vi "Find Center Setup.vi"(0 "Carrier Tray":T1, 1 "Tray Number":dbl format="%#_13g") -> (7 "Assembly Tray Out":T1)   [LabVIEW 2019, in "Assembly Tray.lvclass"]
uses:
  Assembly Tray.lvclass
  Find Tray.ctl
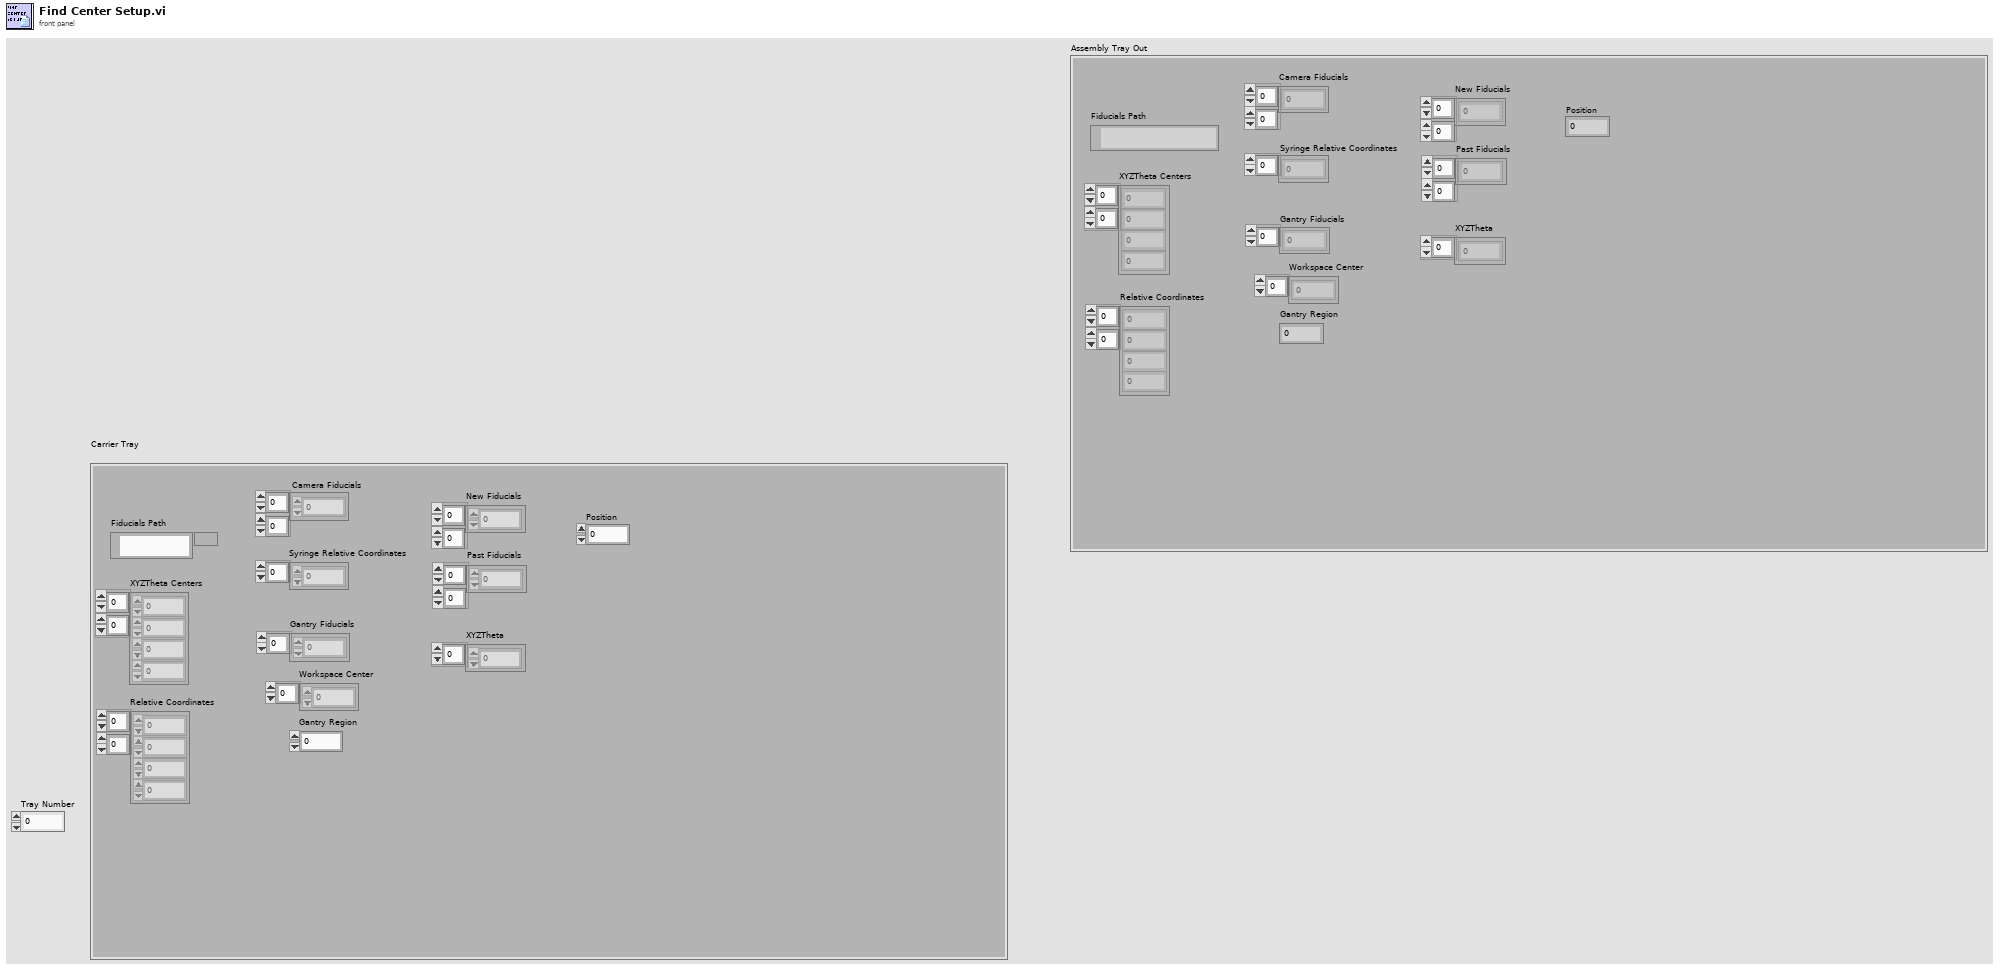
[diagram p1: front panel]
types:
  T1 = typedef "Assembly Tray.lvclass/Find Tray.ctl" = cluster{"Gantry Fiducials":dbl[], "Relative Coordinates":dbl[][], "Camera Fiducials":dbl[][], "XYZTheta Centers":dbl[][], "Workspace Center":dbl[], "Syringe Relative Coordinates":dbl[], "Gantry Region":dbl, "Fiducials Path":path, "New Fiducials":dbl[][], "Past Fiducials":dbl[][], "XYZTheta":dbl[], "Position":i32}
  T2 = typedef "File Paths.ctl" = cluster{"Glue Pattern Folder":path, "Carrier Tray Folder":path, "Pick Up Tool Fixture Folder":path, "Components Folder":path, "Bellows Tool Offset.txt":path, "Pick Up Tool Offset.txt":path, "Dispense Tip Offset.txt":path, "Log Files":path}
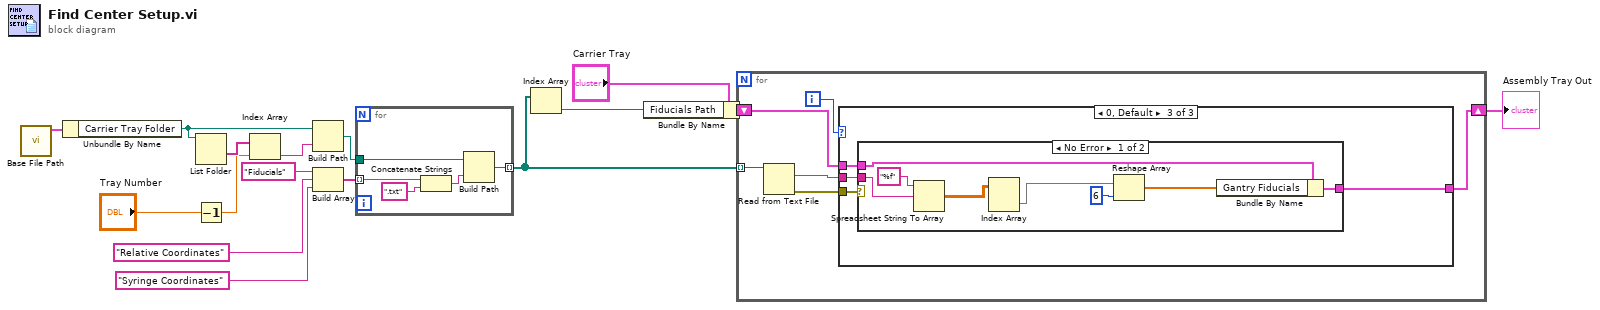
[diagram p0: block diagram]
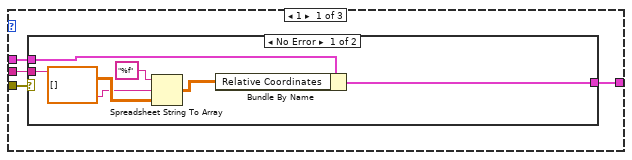
[diagram p2: hidden frame]
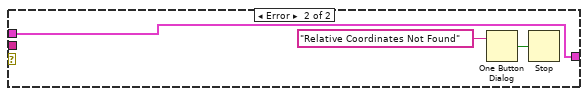
[diagram p3: hidden frame]
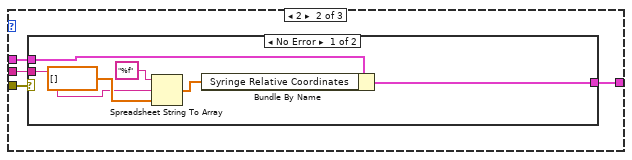
[diagram p4: hidden frame]
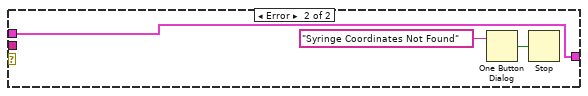
[diagram p5: hidden frame]
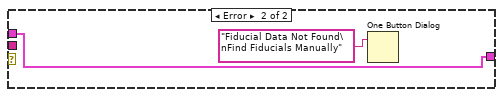
[diagram p6: hidden frame]
diagram:
  n1 = call "Base File Path.vi"() -> ("Paths Out"=w8:T2)  [unwired: 11 in]
  n2 = Unbundle By Name(w8) -> ("Carrier Tray Folder"=w4:path)
  n3 = List Folder(path=w4) -> (folder names=w10:string[])  [unwired: 3 in, 3 out]
  n4 = Decrement(x="Tray Number") -> (x-1=w6:dbl)
  n5 = Index Array(array=w10, index=w6) -> (element=w9:string)
  n6 = Build Path(base path=w4, name or relative path=w9) -> (appended path=w12:path)
  n7 = Build Array("Fiducials" ("format string"), "Relative Coordinates" ("format string"), "Syringe Coordinates" ("element")) -> (w11:string[])
  n8 = for {
    tunnel: w11 -> [w19] mode=indexing
    tunnel: w12 -> [w21]
    tunnel: [w20] -> w2 mode=indexing
    n9 = Concatenate Strings(w19, ".txt" ("string")) -> (w17:string)
    n10 = Build Path(base path=w21, name or relative path=w17) -> (appended path=w20:path)
  }
  n11 = Index Array(array=w2) -> (element=w13:path)  [unwired: 1 in]
  n12 = Bundle By Name(cluster="Carrier Tray", "Fiducials Path"=w13) -> (w16:T1)
  n13 = for {
    tunnel: w2 -> [w26] mode=indexing
    shift-right: [w22] -> w5
    shift-left: w16 -> [w23]
    i -> [w24]
    n14 = Read from Text File(file (use dialog)=w26) -> (text=w27:string, error out=w25:errorcluster)  [unwired: 3 in, 2 out]
    n15 = case shown="0, Default" w24 {
      tunnel: w27 -> [w30 w42 w57]
      tunnel: w25 -> [w31 w43 w56]
      tunnel: w23 -> [w29 w44 w55]
      tunnel: [w28 w41 w54] -> w22
      frame 1 {
        n16 = case shown="No Error" w31 {
          tunnel: w30 -> [w35 _]
          tunnel: [w33 w38] -> w28
          tunnel: w29 -> [w34 w38]
          frame No Error {
            n17 = Spreadsheet String To Array(format string="%f", spreadsheet string=w35, array type (2D Dbl)=dbl[][] []) -> (array=w32:dbl[][])  [unwired: 1 in]
            n18 = Bundle By Name(cluster=w34, "Relative Coordinates"=w32) -> (w33:T1)
          }
          frame Error {
            n19 = One Button Dialog(message="Relative Coordinates Not Found") -> (true=w39:bool)  [unwired: 1 in]
            n20 = Stop(stop? (T)=w39) -> ()
          }
        }
      }
      frame 2 {
        n21 = case shown="No Error" w43 {
          tunnel: w42 -> [w48 _]
          tunnel: [w46 w51] -> w41
          tunnel: w44 -> [w47 w51]
          frame No Error {
            n22 = Spreadsheet String To Array(format string="%f", spreadsheet string=w48, array type (2D Dbl)=dbl[] []) -> (array=w45:dbl[])  [unwired: 1 in]
            n23 = Bundle By Name(cluster=w47, "Syringe Relative Coordinates"=w45) -> (w46:T1)
          }
          frame Error {
            n24 = One Button Dialog(message="Syringe Coordinates Not Found") -> (true=w52:bool)  [unwired: 1 in]
            n25 = Stop(stop? (T)=w52) -> ()
          }
        }
      }
      frame 0, Default {
        n26 = case shown="No Error" w56 {
          tunnel: w57 -> [w64 _]
          tunnel: w55 -> [w62 w66]
          tunnel: [w63 w66] -> w54
          frame No Error {
            n27 = Spreadsheet String To Array(format string="%f", spreadsheet string=w64) -> (array=w59:dbl[][])  [unwired: 2 in]
            n28 = Index Array(array=w59) -> (element=w58:dbl[])  [unwired: 2 in]
            n29 = Reshape Array(w58, 6 ("dimension size")) -> (w61:dbl[])
            n30 = Bundle By Name(cluster=w62, "Gantry Fiducials"=w61) -> (w63:T1)
          }
          frame Error {
            n31 = One Button Dialog(message="Fiducial Data Not Found\nFind Fiducials Manually") -> ()  [unwired: 1 in, 1 out]
          }
        }
      }
    }
  }
  "Assembly Tray Out" <- w5
